vi "myRIO_BRig_RT_dataTrial_LC_Cue1_Triggered_l1.vi"() -> (2 "output_LC_Cue1_Triggered_l1":i32)   [LabVIEW 2014]
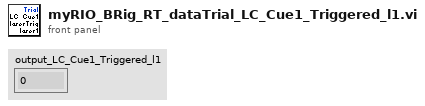
[diagram p1: front panel]
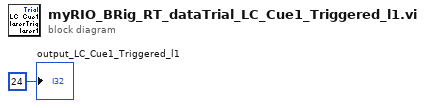
[diagram p0: block diagram]
diagram:
  "output_LC_Cue1_Triggered_l1" <- 24 ("output_iBlock")
